vi "OpenPort.vi"(0 "COM Port (COM1)":T1(ring)=enum."COM2", 2 "BaudRate (19200)":enum32{"9600", "19200", "38400", "57600"}(ring)=enum."19200", 5 "error in (no error)":errorcluster) -> (14 "handle":i32, 19 "error out":errorcluster)   [LabVIEW 2014, in "Sixpack - Driver.lvlib"]
uses:
  Sixpack - Driver.lvlib
  DLL/PackDLL.dll
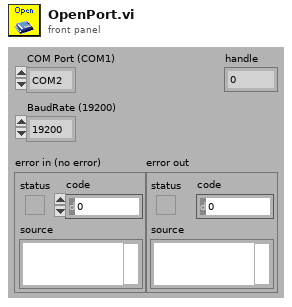
[diagram p1: front panel]
types:
  T1 = enum32{"COM1", "COM2", "COM3", "COM4", "COM5", "COM6", "COM7", "COM8", "COM9"}
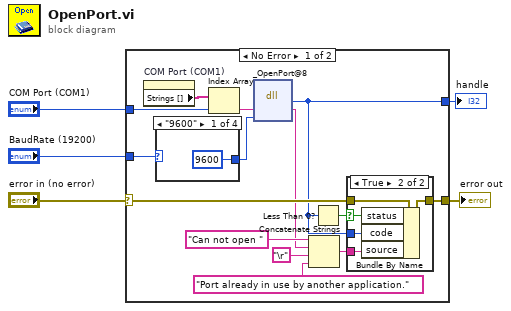
[diagram p0: block diagram]
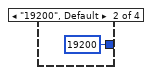
[diagram p3: hidden frame]
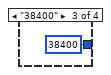
[diagram p4: hidden frame]
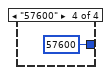
[diagram p5: hidden frame]
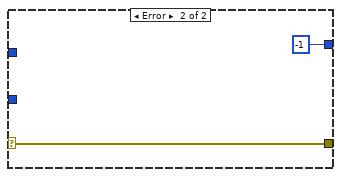
[diagram p6: hidden frame]
diagram:
  n1 = case shown="No Error" "error in (no error)" {
    selector: "error in (no error)" -> [w14 w30]
    tunnel: "COM Port (COM1)" -> [w17 _]
    tunnel: "BaudRate (19200)" -> [w16 _]
    tunnel: [w12 -1 ("handle")] -> w3
    tunnel: [w13 w30] -> w1
    frame No Error {
      n2 = property on="COM Port (COM1)" class="Enum (strict)"() -> ("Strings []"=w18:string[])  [unwired: 2 in, 2 out]
      n3 = case shown="\"9600\"" w16 {
        tunnel: [9600 ("BaudRate") 19200 ("BaudRate") 38400 ("BaudRate") 57600 ("BaudRate")] -> w15
        frame "9600" {
        }
        frame "19200", Default {
        }
        frame "38400" {
        }
        frame "57600" {
        }
      }
      n4 = Index Array(array=w18, index=w17) -> (element=w19:string)
      n5 = dll-call lib="D:/CS-Source/LV2014/GPL/instr.lib/SixPack/PackDLL/DLL/PackDLL.dll" fn="_OpenPort@8" label="OpenPort"("PortName"=w19, "BaudRate"=w15) -> ("handle"=w12:i32, "PortName"=w7:string)  [unwired: 4 in, 2 out]
      n6 = Concatenate Strings("Can not open " ("source"), w7, "\r", "Port already in use by another application." ("source")) -> (w11:string)
      n7 = Less Than 0?(x=w12) -> (x < 0?=w6:bool)
      n8 = case shown="True" w6 {
        selector: w6 -> [_ w21]
        tunnel: w14 -> [w20 w25]
        tunnel: [w20 w24] -> w13
        tunnel: w12 -> [_ w23]
        tunnel: w11 -> [_ w22]
        frame False {
        }
        frame True {
          n9 = Bundle By Name(cluster=w25, "status"=w21, "code"=w23, "source"=w22) -> (w24:errorcluster)
        }
      }
    }
    frame Error {
    }
  }
  "handle" <- w3
  "error out" <- w1
